vi "Is UI Ready.vi"(9 "Logger Running?":bool, 10 "Acquisition Running?":bool, 11 "Settings Editor Running?":bool) -> (3 "Status":string)   [LabVIEW 2019, in "CML UI.lvlib"]
doc: "_____\nBased on DQMH Project Template 6.1.0.94."
uses:
  CML UI.lvlib
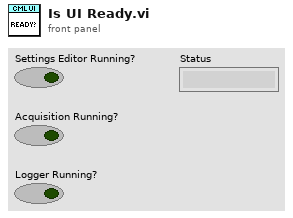
[diagram p1: front panel]
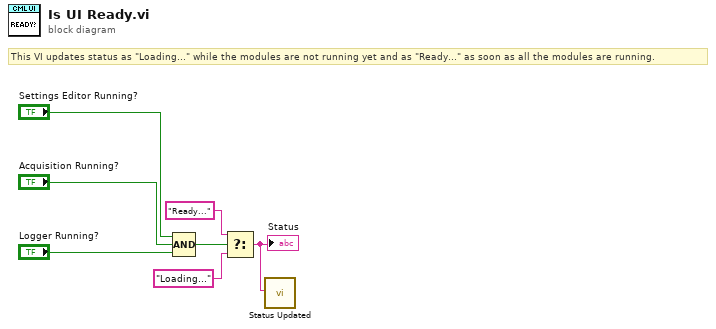
[diagram p0: block diagram]
diagram:
  # "This VI updates status as \"Loading...\" while the modules are not running yet and as \"Ready...\" as soon as all the modules are running."
  n1 = Compound Arithmetic op=AND("Settings Editor Running?", "Acquisition Running?", "Logger Running?") -> (w3:bool)
  n2 = Select(t="Ready...", s=w3, f="Loading...") -> (s? t:f=w7:string)
  "Status" <- w7
  n3 = call "Status Updated.vi"("Status"=w7) -> ()  [unwired: 10 in, 1 out]
